vi "listener.vi"(10 "parameters":T1, 11 "websocket standalone server in":refnum<class "websocket standalone server.lvclass">) -> ()   [LabVIEW 2016, in "websocket standalone server.lvclass"]
uses:
  websocket standalone server.lvclass
  websocket connection parameters.ctl
  websocket standalone server.lvclass/websocket standalone server.ctl
  websocket data packet.ctl
  websocket message type.ctl
  connection handler.vi
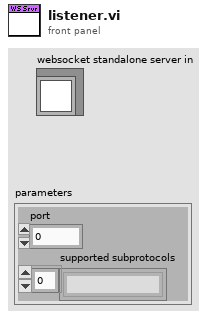
[diagram p1: front panel]
types:
  T1 = typedef "websocket standalone server.lvclass/websocket connection parameters.ctl" = cluster{"port":u16, "supported subprotocols":string[]}
  T2 = typedef "websocket standalone server.lvclass/websocket data packet.ctl" = cluster{"message type":T3, "data":string}
  T3 = typedef "websocket standalone server.lvclass/websocket message type.ctl" = enum16{"UTF8 data", "binary data", "close", "ping", "pong"}
  T4 = typedef "websocket standalone server.lvclass/websocket listener message.ctl" = enum16{"exit", "block socket", "unblock socket"}
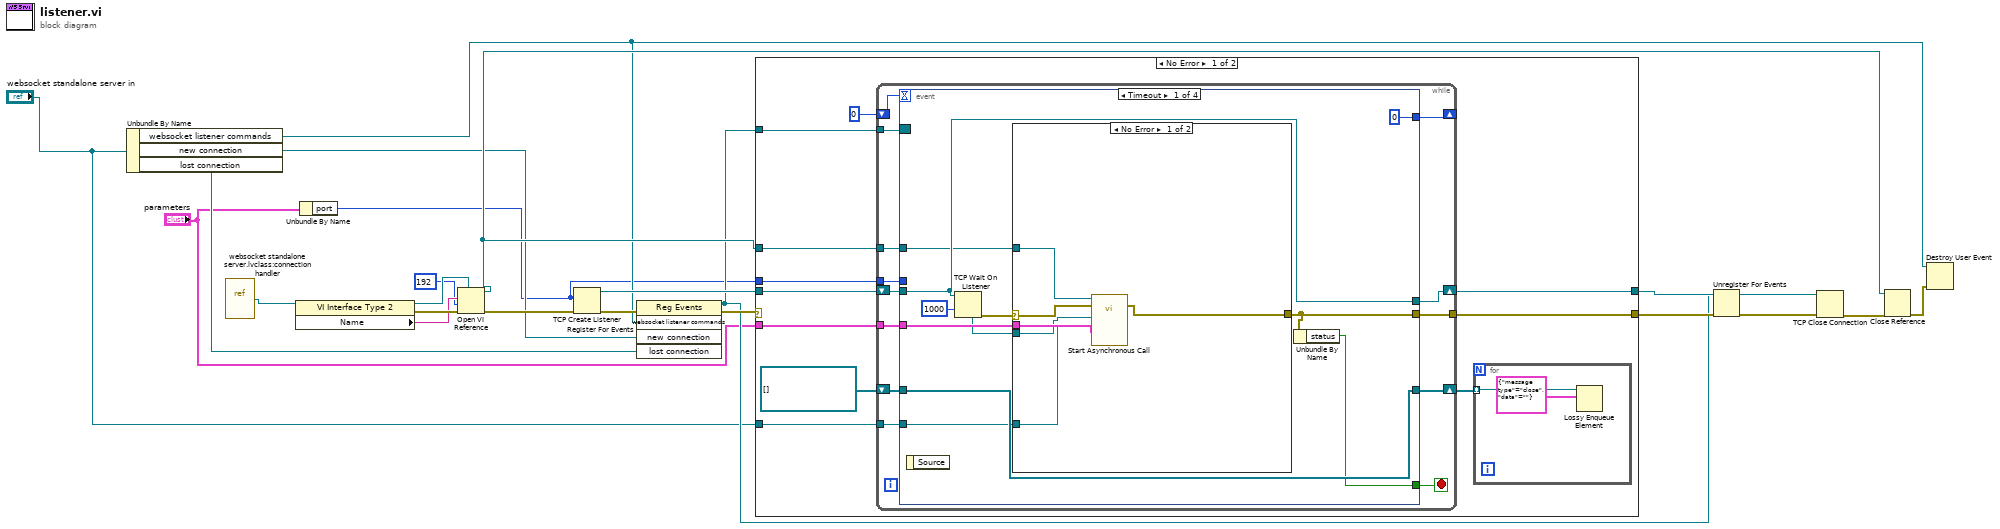
[diagram p0: block diagram]
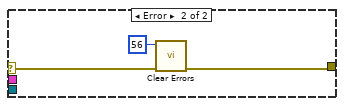
[diagram p2: hidden frame]
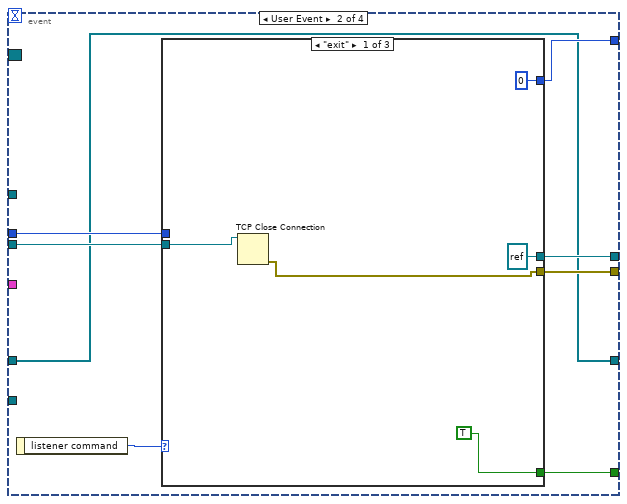
[diagram p3: hidden frame]
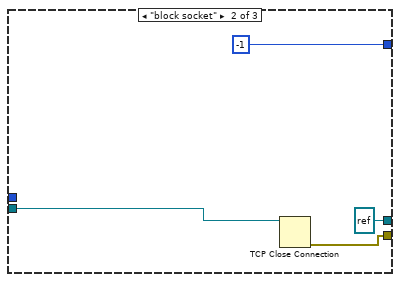
[diagram p4: hidden frame]
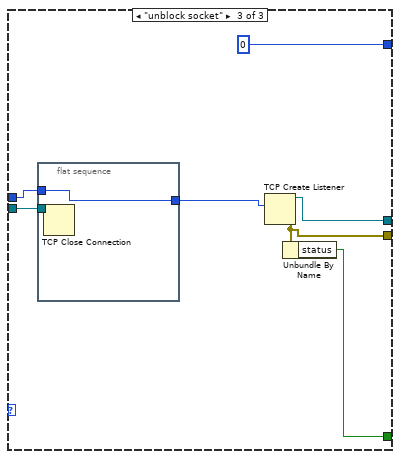
[diagram p5: hidden frame]
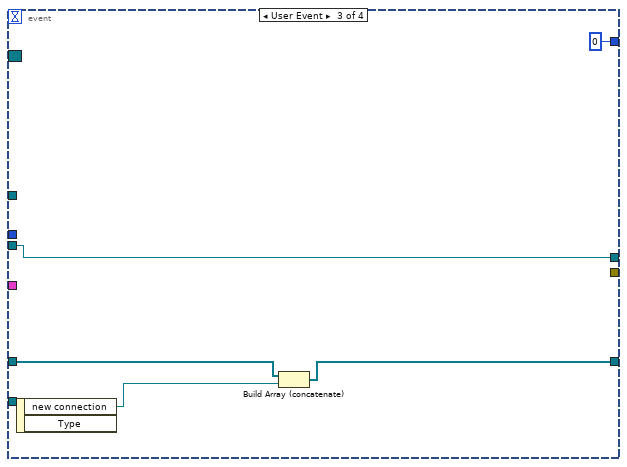
[diagram p6: hidden frame]
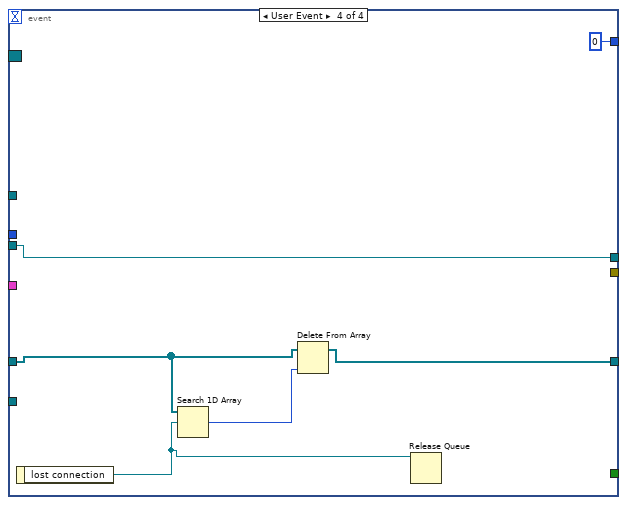
[diagram p7: hidden frame]
diagram:
  n1 = Unbundle By Name("websocket standalone server in") -> ("websocket listener commands"=w7:refnum<user-event>, "new connection"=w6:refnum<user-event>, "lost connection"=w5:refnum<user-event>)
  n2 = vi-ref "websocket standalone server.lvclass:connection handler.vi"() -> (w22:refnum<vi>)
  n3 = property class="VI Interface Type 2"(reference=w22) -> (reference out=w19:refnum<vi>, error out=w21:errorcluster, "Name"=w20:string)  [unwired: 1 in]
  n4 = Unbundle By Name("parameters") -> ("port"=w3:u16)
  n5 = Open VI Reference(type specifier VI Refnum (for type only)=w19, vi path=w20, options=192, error in (no error)=w21) -> (vi reference=w11:refnum<vi>, error out=w17:errorcluster)  [unwired: 2 in]
  n6 = TCP Create Listener(8:w17, 10:w3) -> (0:w16:errorcluster, 3:w14:refnum<k5>)  [unwired: 3 in, 1 out]
  n7 = register-events(error in=w16, w7, w6, w5) -> (reference out=w4:refnum<event-registration>, error out=w9:errorcluster)  [unwired: 1 in]
  n8 = case shown="No Error" w9 {
    selector: w9 -> [_ w106]
    tunnel: [w27 w107] -> w15
    tunnel: w14 -> [w33 w107]
    tunnel: [w25 w106] -> w13
    tunnel: w11 -> [w32 _]
    tunnel: w4 -> [w30 _]
    tunnel: w3 -> [w26 _]
    tunnel: "parameters" -> [w24 _]
    tunnel: "websocket standalone server in" -> [w23 _]
    frame No Error {
      n9 = while {
        shift-right: [w43] -> w27
        shift-left: w33 -> [w48]
        tunnel: w32 -> [w47]
        shift-right: [w45] -> _
        shift-left: 0 -> [w46]
        tunnel: w30 -> [w44]
        shift-right: [w38] -> w28
        shift-left: refnum<queue>[] [] -> [w41]
        tunnel: w26 -> [w40]
        tunnel: [w39] -> w25
        tunnel: w24 -> [w37]
        tunnel: w23 -> [w36]
        stop <- w42 stop-if-true
        n10 = event shown="[0] Timeout" {
          selector: w44 -> [_ _ _ _]
          dyn-events: _ -> [_ _ _ _]
          timeout: w46 -> [_ _ _ _]
          tunnel: w48 -> [w59 w74 w99 w105]
          tunnel: w47 -> [w56 _ _ _]
          tunnel: [0 w73 0 0] -> w45
          tunnel: [w59 w75 w99 w105] -> w43
          tunnel: [w52 w72 _ _] -> w42
          tunnel: w41 -> [w54 w69 w98 w103]
          tunnel: w40 -> [_ w71 _ _]
          tunnel: [w53 w70 _ _] -> w39
          tunnel: [w54 w69 w96 w104] -> w38
          tunnel: w37 -> [w51 _ _ _]
          tunnel: w36 -> [w50 _ _ _]
          event Timeout {
            n11 = event-data() -> ()  [unwired: 1 in, 1 out]
            n12 = TCP Wait On Listener(9:1000 ("timeout ms (wait forever: -1)"), 11:w59) -> (0:w57:errorcluster, 4:w49:refnum<k5>)  [unwired: 2 in, 3 out]
            n13 = case shown="No Error" w57 {
              selector: w57 -> [w65 w68]
              tunnel: w56 -> [w64 _]
              tunnel: [w63 w67] -> w53
              tunnel: w51 -> [w62 _]
              tunnel: w50 -> [w61 _]
              tunnel: w49 -> [w60 _]
              frame No Error {
                n14 = call-by-ref "Start Asynchronous Call"(reference=w64, error in=w65, "parameters"=w62, "websocket standalone server in"=w61, "connection ID"=w60) -> (error out=w63:errorcluster)  [unwired: 9 in, 1 out]
              }
              frame Error {
                n15 = call <vilib>:"Clear Errors.vi"("error in (no error)"=w68, "specific error code to clear (0: all)"=56) -> ("error out"=w67:errorcluster)  [unwired: 4 in, 1 out]
              }
            }
            n16 = Unbundle By Name(w53) -> ("status"=w52:bool)
          }
          event User Event {
            n17 = event-data() -> ("listener command"=w76:T4)  [unwired: 1 in]
            n18 = case shown="\"exit\"" w76 {
              tunnel: [refnum<k5> refnum ("listener ID") refnum<k5> refnum ("listener ID") w88] -> w75
              tunnel: w74 -> [w79 w85 w92]
              tunnel: [0 -1 0] -> w73
              tunnel: [TRUE _ w87] -> w72
              tunnel: w71 -> [_ _ w90]
              tunnel: [w77 w82 w86] -> w70
              frame "exit" {
                n19 = TCP Close Connection(connection ID=w79) -> (error out=w77:errorcluster)  [unwired: 2 in, 1 out]
              }
              frame "block socket" {
                n20 = TCP Close Connection(connection ID=w85) -> (error out=w82:errorcluster)  [unwired: 2 in, 1 out]
              }
              frame "unblock socket" {
                n21 = flat-sequence {
                  tunnel: w92 -> [w94]
                  tunnel: w90 -> [w93]
                  tunnel: [w93] -> w89
                  frame #0 {
                    n22 = TCP Close Connection(connection ID=w94) -> ()  [unwired: 2 in, 2 out]
                  }
                }
                n23 = TCP Create Listener(10:w89) -> (0:w86:errorcluster, 3:w88:refnum<k5>)  [unwired: 4 in, 1 out]
                n24 = Unbundle By Name(w86) -> ("status"=w87:bool)
              }
            }
          }
          event User Event {
            n25 = event-data() -> ("new connection"=w97:refnum<queue>)  [unwired: 1 in, 1 out]
            n26 = Build Array (concatenate)(w98, w97) -> (w96:refnum<queue>[])
          }
          event User Event {
            n27 = event-data() -> ("lost connection"=w101:refnum<queue>)  [unwired: 1 in]
            n28 = Search 1D Array(1D array=w103, element=w101) -> (index of element=w102:i32)  [unwired: 1 in]
            n29 = Delete From Array(array=w103, index=w102) -> (array with subset deleted=w104:refnum<queue>[])  [unwired: 1 in, 1 out]
            n30 = Release Queue(queue=w101) -> ()  [unwired: 2 in, 3 out]
          }
        }
      }
      n31 = for {
        tunnel: w28 -> [w35] mode=indexing
        n32 = Lossy Enqueue Element(queue=w35, element=T2 {"message type"=enum."close", "data"=""}) -> ()  [unwired: 1 in, 4 out]
      }
    }
    frame Error {
    }
  }
  n33 = Unregister For Events(event registration refnum=w4, error in=w13) -> (error out=w8:errorcluster)
  n34 = TCP Close Connection(connection ID=w15, error in (no error)=w8) -> (error out=w12:errorcluster)  [unwired: 1 in, 1 out]
  n35 = Close Reference(reference=w11, error in (no error)=w12) -> (error out=w10:errorcluster)
  n36 = Destroy User Event(user event=w7, error in=w10) -> ()  [unwired: 1 out]
